vi "ZoomToFitModeEnabler.vi"() -> ()   [LabVIEW 2023]
uses:
  <vilib>/vision/Image Controls.llb/IMAQ Image.ctl
panel:
  out "Destination Image":T1(plugin-control)
  out "Source Image":T1(plugin-control)
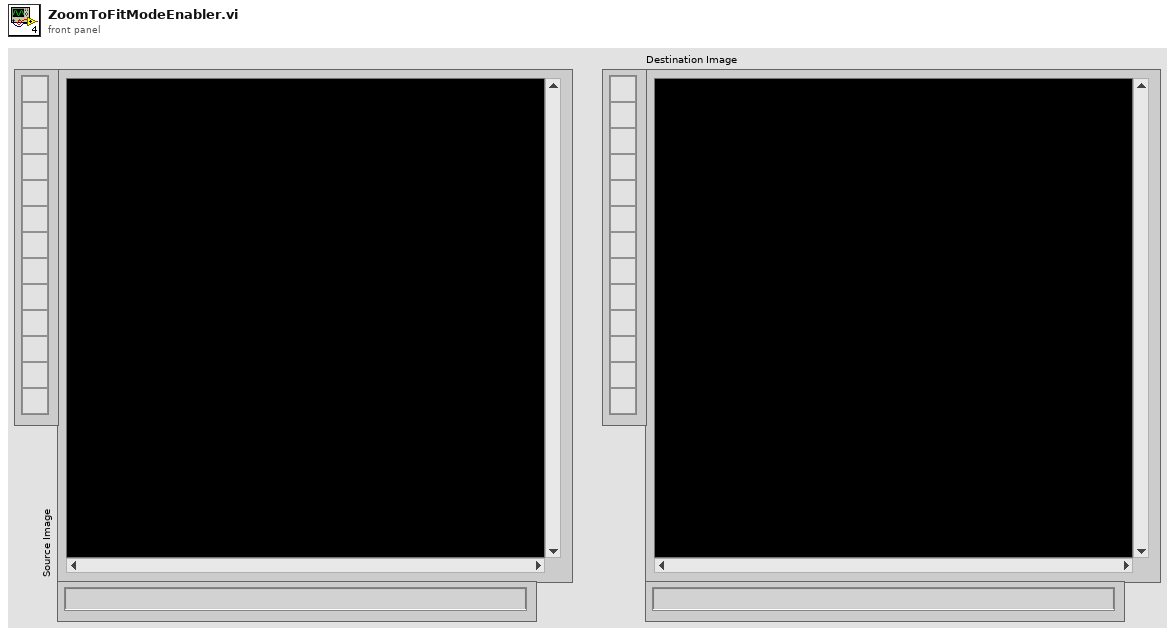
[diagram p1: front panel]
types:
  T1 = typedef "IMAQ Image.ctl" = refnum<image>
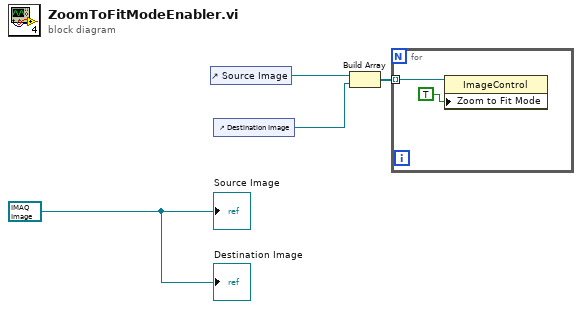
[diagram p0: block diagram]
diagram:
  w1 = T1 refnum ("Source Image")
  n1 = control-ref of="Source Image"() -> (w4:refnum<vi>)
  n2 = control-ref of="Destination Image"() -> (w3:refnum<vi>)
  n3 = Build Array(w4, w3) -> (w2:refnum<vi>[])
  n4 = for {
    tunnel: w2 -> [w6] mode=indexing
    n5 = property class="ImageControl"(reference=w6, "Zoom to Fit Mode"=TRUE) -> ()  [unwired: 1 in, 2 out]
  }
  "Source Image" <- w1
  "Destination Image" <- w1
